vi "Dequeue.vi"(8 "error in":errorcluster) -> (0 "error out":errorcluster, 2 "Data":variant, 3 "State":T1)   [LabVIEW 2018, in "Serial.lvclass"]
uses:
  Serial.lvclass
  State.ctl
  Queue Data.ctl
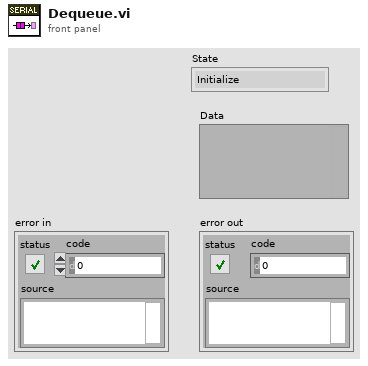
[diagram p1: front panel]
types:
  T1 = typedef "Serial.lvclass/State.ctl" = enum16{"Initialize", "LoadConfig", "Read", "Error", "Exit"}
  T2 = typedef "Serial.lvclass/Queue Data.ctl" = cluster{"State":T1, "Data":variant}
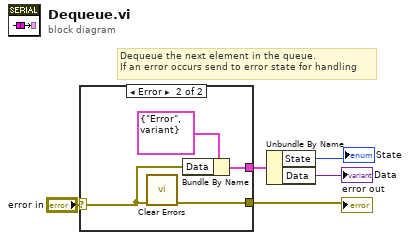
[diagram p0: block diagram]
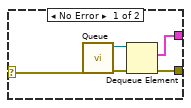
[diagram p2: hidden frame]
diagram:
  # "Dequeue the next element in the queue. \nIf an error occurs send to error state for handling"
  n1 = case shown="Error" "error in" {
    selector: "error in" -> [w10 w12]
    tunnel: [w8 w14] -> w2
    tunnel: [w6 w11] -> w3
    frame No Error {
      n2 = call "Queue.vi"("error in"=w10) -> ("error out"=w9:errorcluster, "queue out"=w7:refnum<queue>)  [unwired: 9 in]
      n3 = Dequeue Element(queue=w7, error in (no error)=w9) -> (element=w6:T2, error out=w8:errorcluster)  [unwired: 1 in, 2 out]
    }
    frame Error {
      n4 = call <vilib>:"Clear Errors.vi"("error in (no error)"=w12) -> ("error out"=w14:errorcluster)  [unwired: 5 in, 1 out]
      n5 = Bundle By Name(cluster=T2 {"State"=enum."Error", "Data"=variant}, "Data"=w12) -> (w11:T2)
    }
  }
  "error out" <- w2
  n6 = Unbundle By Name(w3) -> ("State"=→"State":T1, "Data"=→"Data":variant)
